vi "msc_zerowe.vi"(8 "d":dbl, 9 "c":dbl, 10 "b":dbl, 11 "a":dbl) -> (0 "Ilość pierwiastków rzeczywistych":i16, 1 "x3":cdb, 2 "x2":cdb, 3 "x1":cdb)   [LabVIEW 2020]
doc: "Obliczanie pierwiastków wielomianu 3 stopnia z użyciem postaci kanonicznej metodą analityczną"
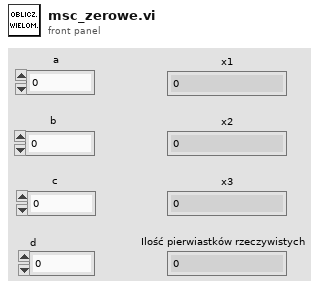
[diagram p1: front panel]
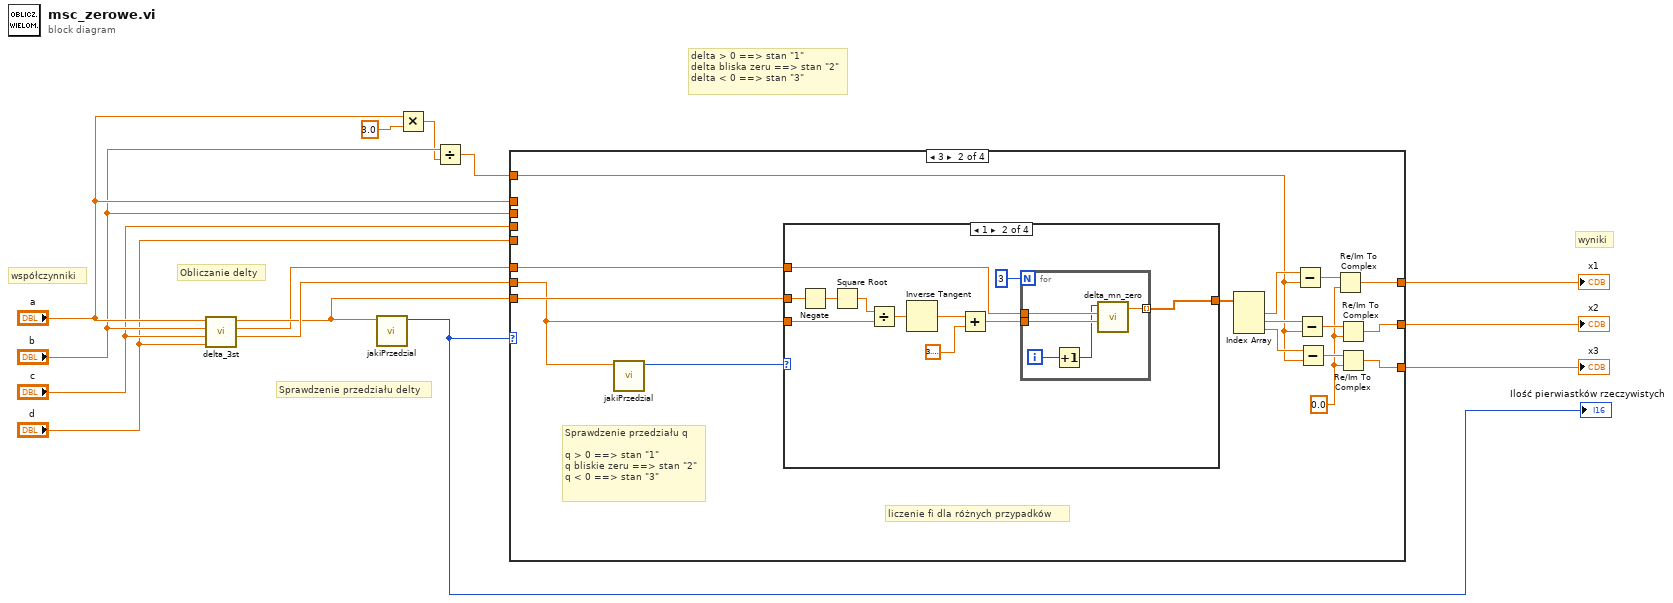
[diagram p0: block diagram]
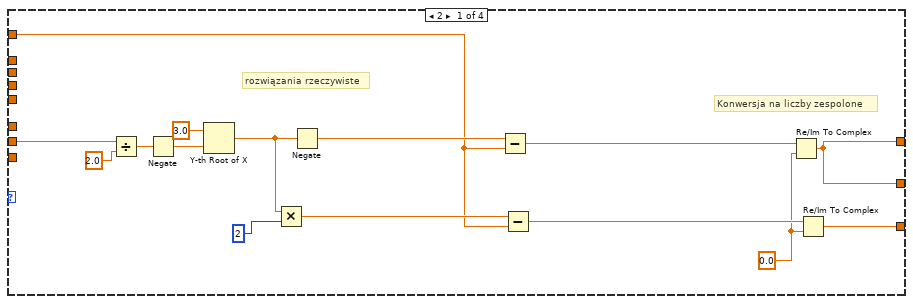
[diagram p2: hidden frame]
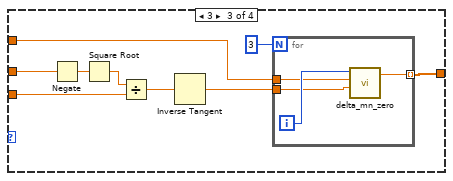
[diagram p4: hidden frame]
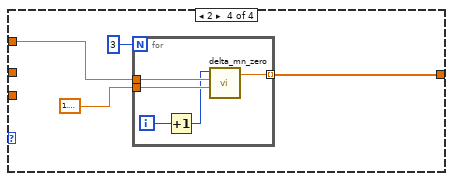
[diagram p5: hidden frame]
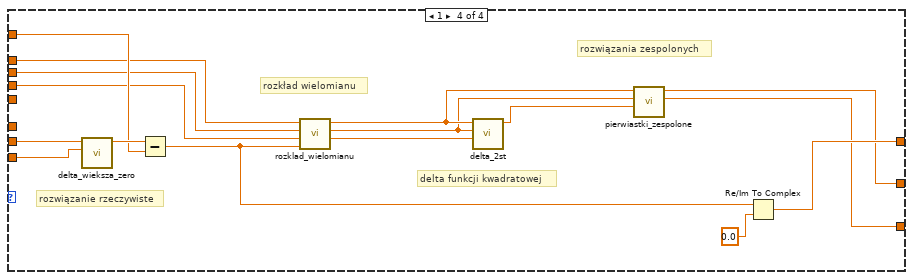
[diagram p7: hidden frame]
diagram:
  # "delta > 0 ==> stan \"1\"\ndelta bliska zeru ==> stan \"2\"\ndelta < 0 ==> stan \"3\""
  # "wyniki"
  # "Sprawdzenie przedziału delty"
  # "Obliczanie delty"
  # "współczynniki"
  n1 = call "delta_3st.vi"("d"="d", "c"="c", "b"="b", "a"="a") -> ("q"=w4:dbl, "p"=w1:dbl, "Delta trzeciego stopnia"=w3:dbl)  [unwired: 5 in]
  n2 = call "jakiPrzedzial.vi"("wejscie"=w3) -> ("selector"=w2:i16)  [unwired: 10 in]
  "Ilość pierwiastków rzeczywistych" <- w2
  n3 = Multiply(x="a", y=3.0) -> (x*y=w6:dbl)
  n4 = Divide(x="b", y=w6) -> (x/y=w7:dbl)
  n5 = case shown="3" w2 {
    tunnel: w3 -> [_ w45 _ w98]
    tunnel: w1 -> [_ w43 _ _]
    tunnel: w4 -> [w27 w30 _ w99]
    tunnel: "a" -> [_ _ _ w95]
    tunnel: "b" -> [_ _ _ w94]
    tunnel: "c" -> [_ _ _ w93]
    tunnel: "d" -> [_ _ _ _]
    tunnel: w7 -> [w20 w38 _ w96]
    tunnel: [w16 w35 _ w84] -> w9
    tunnel: [w16 w33 _ w86] -> w8
    tunnel: [w15 w32 _ w85] -> w10
    frame 2 {
      w17 = 0.0 ("y")
      # "Konwersja na liczby zespolone"
      # "rozwiązania rzeczywiste"
      n6 = Divide(x=w27, y=2.0) -> (x/y=w25:dbl)
      n7 = Negate(x=w25) -> (-x=w24:dbl)
      n8 = Y-th Root of X(1:w24, 2:3.0 ("y")) -> (0:w23:dbl)
      n9 = Multiply(x=w23, y=i16 2) -> (x*y=w21:dbl)
      n10 = Negate(x=w23) -> (-x=w22:dbl)
      n11 = Subtract(x=w22, y=w20) -> (x-y=w18:dbl)
      n12 = Subtract(x=w21, y=w20) -> (x-y=w19:dbl)
      n13 = Re/Im To Complex(1:w17, 2:w18) -> (0:w16:cdb)
      n14 = Re/Im To Complex(1:w17, 2:w19) -> (0:w15:cdb)
    }
    frame 3 {
      w31 = 0.0 ("y")
      # "liczenie fi dla różnych przypadków"
      # "Sprawdzenie przedziału q\n\nq > 0 ==> stan \"1\"\nq bliskie zeru ==> stan \"2\"\nq < 0 ==> stan \"3\""
      n15 = call "jakiPrzedzial.vi"("wejscie"=w30) -> ("selector"=w44:i16)  [unwired: 10 in]
      n16 = case shown="1" w44 {
        tunnel: w45 -> [_ w56 w67 _]
        tunnel: w30 -> [_ w53 w66 _]
        tunnel: w43 -> [_ w49 w64 w77]
        tunnel: [_ w46 w62 w75] -> w42
        frame 0, Default {
        }
        frame 1 {
          n17 = Negate(x=w56) -> (-x=w55:dbl)
          n18 = Square Root(x=w55) -> (sqrt(x)=w54:dbl)
          n19 = Divide(x=w54, y=w53) -> (x/y=w52:dbl)
          n20 = Inverse Tangent(1:w52) -> (0:w51:dbl)
          n21 = Add(x=w51, y=3.141592653589793) -> (x+y=w48:dbl)
          n22 = for {
            N: 3 -> [_]
            tunnel: w49 -> [w61]
            tunnel: w48 -> [w60]
            tunnel: [w59] -> w46 mode=indexing
            i -> [w58]
            n23 = Increment(x=w58) -> (x+1=w57:i32)
            n24 = call "delta_mn_zero.vi"("fi"=w60, "p"=w61, "k"=w57) -> ("y"=w59:dbl)  [unwired: 8 in]
          }
        }
        frame 3 {
          n25 = Negate(x=w67) -> (-x=w70:dbl)
          n26 = Square Root(x=w70) -> (sqrt(x)=w69:dbl)
          n27 = Divide(x=w69, y=w66) -> (x/y=w68:dbl)
          n28 = Inverse Tangent(1:w68) -> (0:w63:dbl)
          n29 = for {
            N: 3 -> [_]
            tunnel: [w74] -> w62 mode=indexing
            tunnel: w64 -> [w72]
            tunnel: w63 -> [w71]
            i -> [w73]
            n30 = call "delta_mn_zero.vi"("fi"=w71, "p"=w72, "k"=w73) -> ("y"=w74:dbl)  [unwired: 8 in]
          }
        }
        frame 2 {
          n31 = for {
            N: 3 -> [_]
            tunnel: w77 -> [w83]
            tunnel: 1.5707963267948966 -> [w82]
            tunnel: [w81] -> w75 mode=indexing
            i -> [w80]
            n32 = Increment(x=w80) -> (x+1=w79:i32)
            n33 = call "delta_mn_zero.vi"("fi"=w82, "p"=w83, "k"=w79) -> ("y"=w81:dbl)  [unwired: 8 in]
          }
        }
      }
      n34 = Index Array(array=w42) -> (element #1=w39:dbl, element #2=w40:dbl, element #3=w41:dbl)  [unwired: 3 in]
      n35 = Subtract(x=w39, y=w38) -> (x-y=w34:dbl)
      n36 = Subtract(x=w40, y=w38) -> (x-y=w36:dbl)
      n37 = Subtract(x=w41, y=w38) -> (x-y=w37:dbl)
      n38 = Re/Im To Complex(1:w31, 2:w34) -> (0:w33:cdb)
      n39 = Re/Im To Complex(1:w31, 2:w36) -> (0:w35:cdb)
      n40 = Re/Im To Complex(1:w31, 2:w37) -> (0:w32:cdb)
    }
    frame 0, Default {
    }
    frame 1 {
      # "rozwiązania zespolonych"
      # "delta funkcji kwadratowej"
      # "rozkład wielomianu"
      # "rozwiązanie rzeczywiste"
      n41 = call "delta_wieksza_zero.vi"("delta"=w98, "q"=w99) -> ("y0"=w97:dbl)  [unwired: 9 in]
      n42 = Subtract(x=w97, y=w96) -> (x-y=w88:dbl)
      n43 = call "rozklad_wielomianu.vi"("x0"=w88, "c"=w93, "b"=w94, "a"=w95) -> ("cp"=w92:dbl, "bp"=w89:dbl, "ap"=w90:dbl)  [unwired: 5 in]
      n44 = call "delta_2st.vi"("c"=w92, "b"=w89, "a"=w90) -> ("Delta drugiego stopnia"=w91:dbl)  [unwired: 8 in]
      n45 = call "pierwiastki_zespolone.vi"("delta"=w91, "bp"=w89, "ap"=w90) -> ("x2"=w85:cdb, "x1"=w84:cdb)  [unwired: 7 in]
      n46 = Re/Im To Complex(1:0.0 ("y"), 2:w88) -> (0:w86:cdb)
    }
  }
  "x3" <- w10
  "x2" <- w9
  "x1" <- w8
